vi "Test STOMP Subscribe.vi"() -> ()   [LabVIEW 2017]
uses:
  Typedefs/Type_AckHeader.ctl
  STOMP.lvclass
panel:
  out "stomp error msg":errorcluster
  out "Body":string
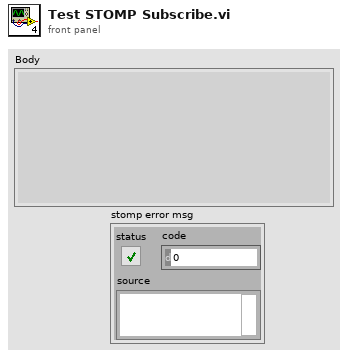
[diagram p1: front panel]
types:
  T1 = typedef "LabVIEW STOMP.lvlib/STOMP.lvclass/Type_AckHeader.ctl" = enum16{"auto", "client", "client-individual"}
  T2 = typedef "LabVIEW STOMP.lvlib/STOMP.lvclass/Type_ServerFrame.ctl" = cluster{"Type":T3, "Headers":cluster{"Header":string, "Value":string}[], "Body":string}
  T3 = typedef "LabVIEW STOMP.lvlib/STOMP.lvclass/Type_ServerFrameType.ctl" = enum16{"Undefined", "MESSAGE", "CONNECTED", "RECEIPT", "ERROR"}
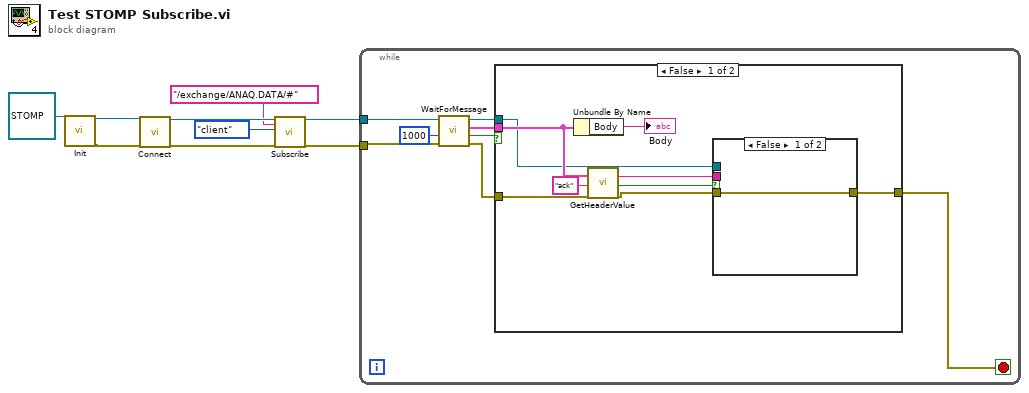
[diagram p0: block diagram]
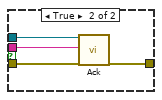
[diagram p2: hidden frame]
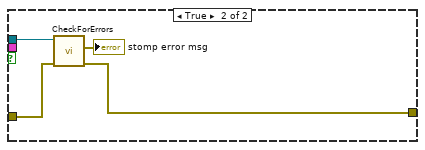
[diagram p3: hidden frame]
diagram:
  n1 = call "Init.vi"("STOMP in"=refnum<class "STOMP.lvclass"> refnum) -> ("STOMP out"=w9:refnum<class "STOMP.lvclass">, "error out"=w8:errorcluster)  [unwired: 17 in]
  n2 = call "Connect.vi"("STOMP in"=w9, "error in"=w8) -> ("STOMP out"=w7:refnum<class "STOMP.lvclass">, "error out"=w6:errorcluster)  [unwired: 16 in]
  n3 = call-dynamic "Subscribe.vi"("STOMP in"=w7, "Destination"="/exchange/ANAQ.DATA/#", "ack"=Type_AckHeader."client", "error in (no error)"=w6) -> ("STOMP out"=w3:refnum<class "STOMP.lvclass">, "error out"=w2:errorcluster)  [unwired: 13 in, 1 out]
  n4 = while {
    tunnel: w3 -> [w10]
    tunnel: w2 -> [w17]
    stop <- w11 stop-if-true
    n5 = call-dynamic "WaitForMessage.vi"("error in (no error)"=w17, "timeout in ms (10000)"=1000, "STOMP in"=w10) -> ("error out"=w12:errorcluster, "timed out?"=w15:bool, "message"=w14:T2, "STOMP out"=w13:refnum<class "STOMP.lvclass">)  [unwired: 5 in]
    n6 = case shown="False" w15 {
      tunnel: w14 -> [w25 _]
      tunnel: w13 -> [w23 w35]
      tunnel: w12 -> [w20 w34]
      tunnel: [w18 w33] -> w11
      frame False {
        n7 = Unbundle By Name(w25) -> ("Body"=→"Body":string)
        n8 = call "GetHeaderValue.vi"("Server Frame"=w25, "Header Name"="ack", "error in"=w20) -> ("Value"=w22:string, "Found?"=w21:bool, "error out"=w19:errorcluster)  [unwired: 14 in]
        n9 = case shown="False" w21 {
          tunnel: w23 -> [_ w31]
          tunnel: w22 -> [_ w30]
          tunnel: w19 -> [w27 w29]
          tunnel: [w27 w28] -> w18
          frame False {
          }
          frame True {
            n10 = call-dynamic "Ack.vi"("STOMP in"=w31, "ack id"=w30, "error in (no error)"=w29) -> ("error out"=w28:errorcluster)  [unwired: 15 in, 1 out]
          }
        }
      }
      frame True {
        n11 = call-dynamic "CheckForErrors.vi"("error in (no error)"=w34, "STOMP in"=w35) -> ("error out"=w33:errorcluster, "stomp error msg"=→"stomp error msg":errorcluster)  [unwired: 7 in, 1 out]
      }
    }
  }
